vi "题目4.vi"() -> ()   [LabVIEW 2017]
uses:
  <vilib>/measure/NI_MABase.lvlib
panel:
  out "大小":i32
  out "最小值":dbl
  out "dt":dbl
  out "Y":dbl[](array[numeric])
  in  "采样信息":cluster{"Fs":dbl, "#s":dbl}={"Fs"=1000.0, "#s"=1000.0} {"Fs" format="%.2p"}
  in  "相位":dbl format="%.2p"
  in  "幅值":dbl=1.0 format="%.2p"
  in  "频率":dbl=10.0 format="%.2p"
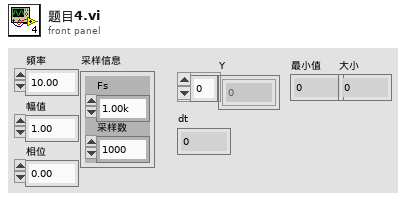
[diagram p1: front panel]
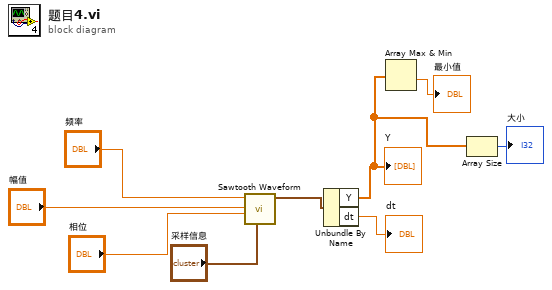
[diagram p0: block diagram]
diagram:
  n1 = call <vilib>:"Sawtooth Waveform.vi"("sampling info"="采样信息", "phase"="相位", "amplitude"="幅值", "frequency"="频率") -> ("signal out"=w5:waveform(dbl))  [unwired: 6 in, 1 out]
  n2 = Unbundle By Name(w5) -> ("Y"=w2:dbl[], "dt"=→"dt":dbl)
  "Y" <- w2
  n3 = Array Max & Min(array=w2) -> (min value=→"最小值":dbl)  [unwired: 3 out]
  n4 = Array Size(array=w2) -> (size(s)=→"大小":i32)
